vi "Speak text ASYNC.vi"(1 "vi path":path=path "C:/Users/Paul Nathan/Desktop/Text to speech async.vi", 2 "Text to speak":string="Warning, Allan Wells will give you a thick ear. Please proceed with caution.") -> (0 "error out":errorcluster)   [LabVIEW 2013]
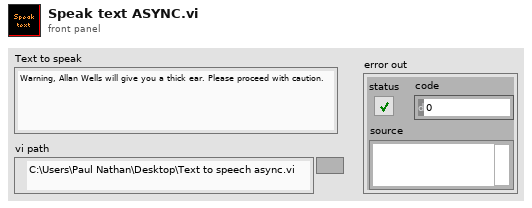
[diagram p1: front panel]
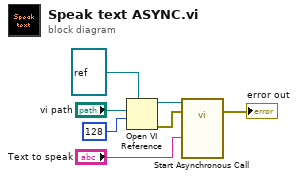
[diagram p0: block diagram]
diagram:
  n1 = Open VI Reference(type specifier VI Refnum (for type only)=refnum<vi> refnum, vi path="vi path", options=128) -> (vi reference=w6:refnum<vi>, error out=w5:errorcluster)  [unwired: 3 in]
  n2 = call-by-ref "Start Asynchronous Call"(reference=w6, error in=w5, "Text to speak"="Text to speak") -> (error out=→"error out":errorcluster)  [unwired: 1 out]
